vi "TH_RS232_Exit.vi"(4 "Array":errorcluster[](array[cluster]), 7 "COMports":refnum<visa-resource-name>[](array[refnum])) -> ()   [LabVIEW 2014]
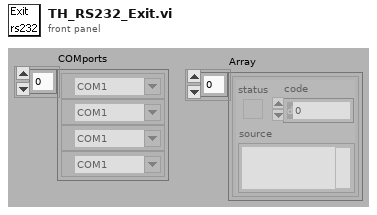
[diagram p1: front panel]
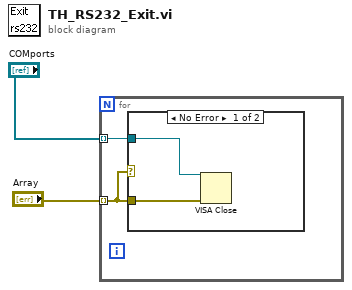
[diagram p0: block diagram]
diagram:
  n1 = for {
    tunnel: "COMports" -> [w4] mode=indexing
    tunnel: "Array" -> [w3] mode=indexing
    n2 = case shown="No Error" w3 {
      tunnel: w3 -> [w6 _]
      tunnel: w4 -> [w5 _]
      frame No Error {
        n3 = VISA Close(VISA resource name=w5, error in (no error)=w6) -> ()  [unwired: 1 out]
      }
      frame Error {
      }
    }
  }
